vi "Fire_BurstPuls.vi"(1 "error in":errorcluster) -> (0 "error out":errorcluster)   [LabVIEW 2016]
uses:
  Utility/Global_Laser.vi
  Program Files (x86)/OPOTEK_DLL/OPOTEK.dll
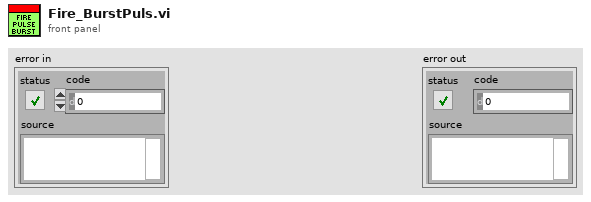
[diagram p1: front panel]
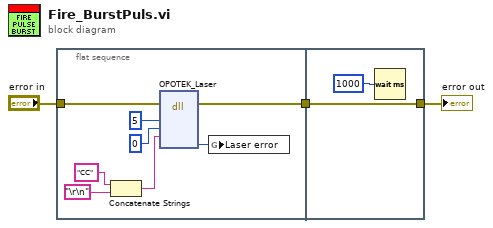
[diagram p0: block diagram]
diagram:
  n1 = flat-sequence {
    tunnel: [w6] -> w1
    tunnel: "error in" -> [w4]
    tunnel: [w13] -> w2
    tunnel: w1 -> [w13]
    frame #0 {
      n2 = Concatenate Strings("CC", "\r\n") -> (w11:string)
      n3 = dll-call lib="C:/Program Files (x86)/OPOTEK_DLL/OPOTEK.dll" fn="OPOTEK_Laser"(error in=w4, "action"=i8 5, "parameter"=i16 0, "stringToSend"=w11) -> (error out=w6:errorcluster, "error_Code"=w7:i32)  [unwired: 7 in, 1 out]
      n4 = global write "Global_Laser.vi" "Laser error"(w7) -> ()
    }
    frame #1 {
      n5 = Wait (ms)(milliseconds to wait=u32 1000 ("Zu wartende ms")) -> ()  [unwired: 1 out]
    }
  }
  "error out" <- w2
